vi "Guitar Tuner.vi"() -> ()   [LabVIEW 2020]
uses:
  <vilib>/Analysis/2dsp.llb/Real FFT.vi
  <vilib>/Analysis/NI_AALPro.lvlib
panel:
  out "Freq":dbl
  out "Amp":dbl
  out "Waveform Graph 8":dbl[](graph)
  out "Waveform Graph 5":cluster{dbl, dbl, dbl[]}(graph)
  in  "stop 5":bool
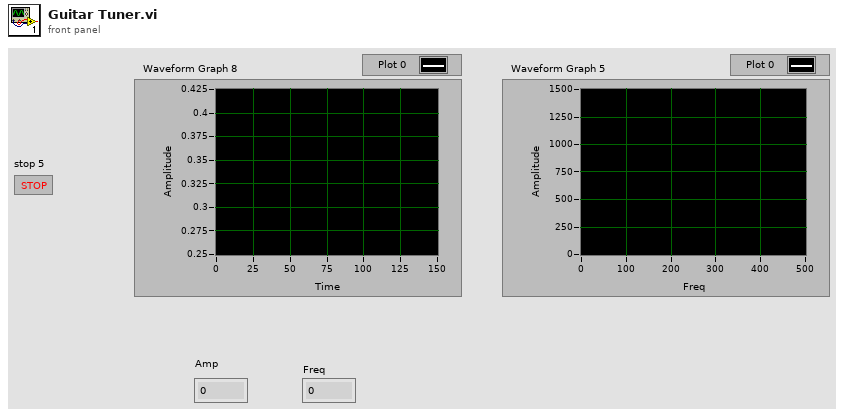
[diagram p1: front panel]
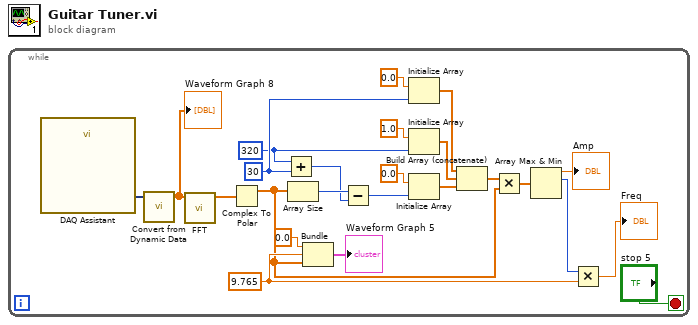
[diagram p0: block diagram]
diagram:
  n1 = while {
    stop <- "stop 5" stop-if-true
    w4 = 320
    w11 = 30
    w15 = 9.765
    n2 = call "DAQ Assistant"() -> ("data"=w21:dynamicdata)  [unwired: 17 in, 2 out]
    n3 = call "Convert from Dynamic Data"("Dynamic Data Type"=w21) -> ("Array"=w23:dbl[])  [unwired: 3 in]
    "Waveform Graph 8" <- w23
    n4 = call-poly <vilib>:"FFT.vi"("X"=w23) -> ("FFT {X}"=w20:cdb[])  [unwired: 9 in, 1 out]
    n5 = Complex To Polar(r * e^(i*theta)=w20) -> (r=w13:dbl[])  [unwired: 1 out]
    n6 = Add(x=w4, y=w11) -> (x+y=w5:i32)
    n7 = Array Size(array=w13) -> (size(s)=w12:i32)
    n8 = Bundle(0.0, w15, w13) -> (→"Waveform Graph 5":cluster{dbl, dbl, dbl[]})  [unwired: 1 in]
    n9 = Subtract(x=w12, y=w5) -> (x-y=w3:i32)
    n10 = Initialize Array(0.0 ("element"), w11) -> (w9:dbl[])
    n11 = Initialize Array(1.0, w4) -> (w8:dbl[])
    n12 = Initialize Array(0.0, w3) -> (w1:dbl[])
    n13 = Build Array (concatenate)(w9, w8, w1) -> (w6:dbl[])
    n14 = Multiply(x=w6, y=w13) -> (x*y=w7:dbl[])
    n15 = Array Max & Min(array=w7) -> (max value=→"Amp":dbl, max index (indices)=w16:i32)  [unwired: 2 out]
    n16 = Multiply(x=w16, y=w15) -> (x*y=→"Freq":dbl)
  }
